vi "Vision Distance.vi"(3 "Horizontal Distance":dbl) -> (1 "Vision Distance":dbl)   [LabVIEW 2015]
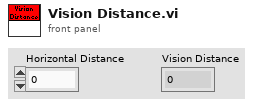
[diagram p1: front panel]
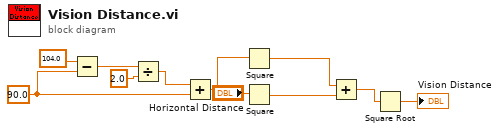
[diagram p0: block diagram]
diagram:
  w2 = 90.0 ("Maximum Goal Height(in)")
  n1 = Subtract(x=104.0 ("Maximum Goal Height(in)"), y=w2) -> (x-y=w4:dbl)
  n2 = Divide(x=w4, y=2.0) -> (x/y=w3:dbl)
  n3 = Add(x=w3, y=w2) -> (x+y=w6:dbl)
  n4 = Square(x=w6) -> (x^2=w10:dbl)
  n5 = Square(x="Horizontal Distance") -> (x^2=w9:dbl)
  n6 = Add(x=w10, y=w9) -> (x+y=w8:dbl)
  n7 = Square Root(x=w8) -> (sqrt(x)=→"Vision Distance":dbl)
